vi "CopyDlls.vi"(11 "Destination Path":path) -> ()   [LabVIEW 2017]
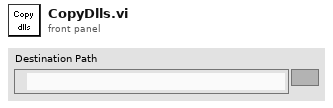
[diagram p1: front panel]
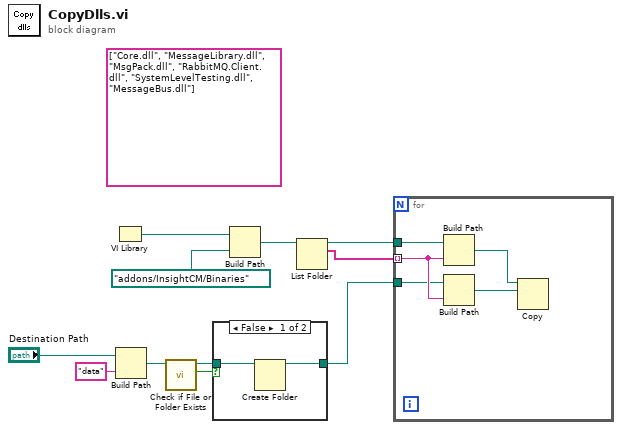
[diagram p0: block diagram]
diagram:
  (unwired) string[] ["Core.dll", "MessageLibrary.dll", "MsgPack.dll", "RabbitMQ.Client.dll", "SystemLevelTesting.dll", "MessageBus.dll"]
  n1 = VI Library() -> (path=w9:path)
  n2 = Build Path(base path="Destination Path", name or relative path="data") -> (appended path=w4:path)
  n3 = call <vilib>:"Check if File or Folder Exists.vi"("path"=w4) -> ("file or folder exists?"=w1:bool, "dup path"=w2:path)  [unwired: 8 in, 1 out]
  n4 = case shown="False" w1 {
    tunnel: [w12 w14] -> w3
    tunnel: w2 -> [w13 w14]
    frame False {
      n5 = Create Folder(path (use dialog)=w13) -> (created path=w12:path)  [unwired: 2 in, 2 out]
    }
    frame True {
    }
  }
  n6 = Build Path(base path=w9, name or relative path=path "addons/InsightCM/Binaries" ("Destination Path")) -> (appended path=w7:path)
  n7 = List Folder(path=w7) -> (path out=w6:path, filenames=w5:string[])  [unwired: 3 in, 2 out]
  n8 = for {
    tunnel: w6 -> [w19]
    tunnel: w5 -> [w16] mode=indexing
    tunnel: w3 -> [w15]
    n9 = Build Path(base path=w19, name or relative path=w16) -> (appended path=w18:path)
    n10 = Build Path(base path=w15, name or relative path=w16) -> (appended path=w17:path)
    n11 = Copy(10:w17, 11:w18) -> ()  [unwired: 3 in, 3 out]
  }
